vi "AB_1200_1100_Project_Destinations.vi"(6 "ProjectPath":path, 7 "action":T3, 8 "error in (no error)":errorcluster, 9 "index":i32, 10 "data in":T2, 11 "buildObject":T1) -> (0 "error out":errorcluster, 1 "index out":i32, 2 "data out":T2, 3 "buildObject out":T1)   [LabVIEW 2020]
doc: "Reads and writes the data to the object property bag."
uses:
  <resource>/Framework/Providers/API/ItemRef.ctl
  <vilib>/AppBuilder/RW_Project/AB_RW_Project_PropBag_Action.ctl
  <vilib>/AppBuilder/AB_Relative_Path_Type.ctl
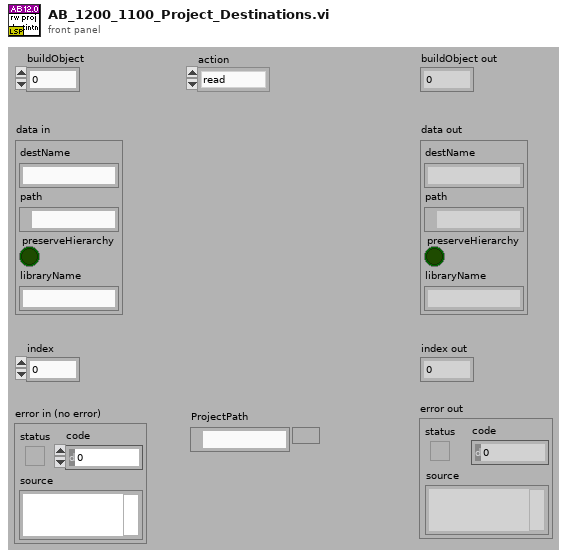
[diagram p1: front panel]
types:
  T1 = typedef "ItemRef.ctl" = u64
  T2 = cluster{"destName":string, "path":path, "preserveHierarchy":bool, "libraryName":string}
  T3 = typedef "AB_RW_Project_PropBag_Action.ctl" = enum16{"read", "write", "clear", "readPrevious", "writePrevious", "clearPrevious"}
  T4 = typedef "AB_Relative_Path_Type.ctl" = enum16{"<none>", "relativeToCommon", "relativeToAppDir", "relativeToProject"}
  T5 = typedef "AB_820_850_Relative_Path_Type.ctl" = enum16{"<none>", "relativeToCommon", "relativeToAppDir"}
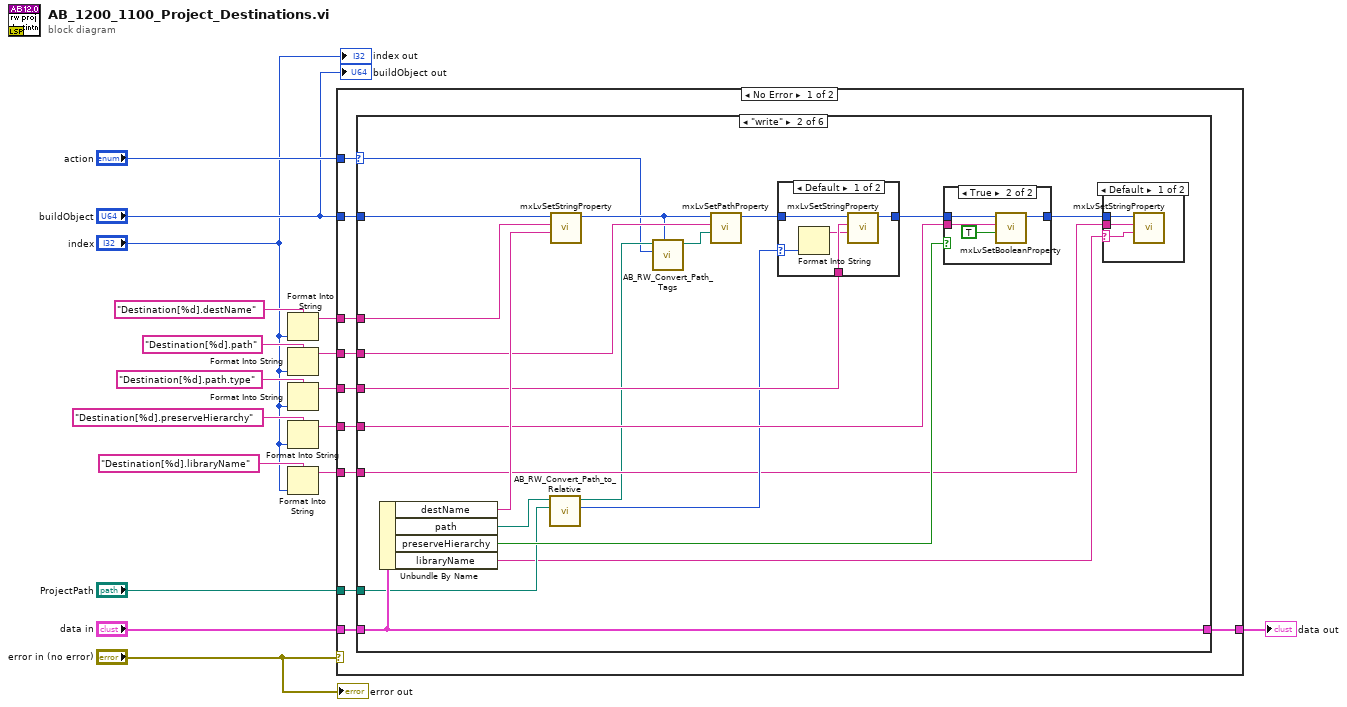
[diagram p0: block diagram]
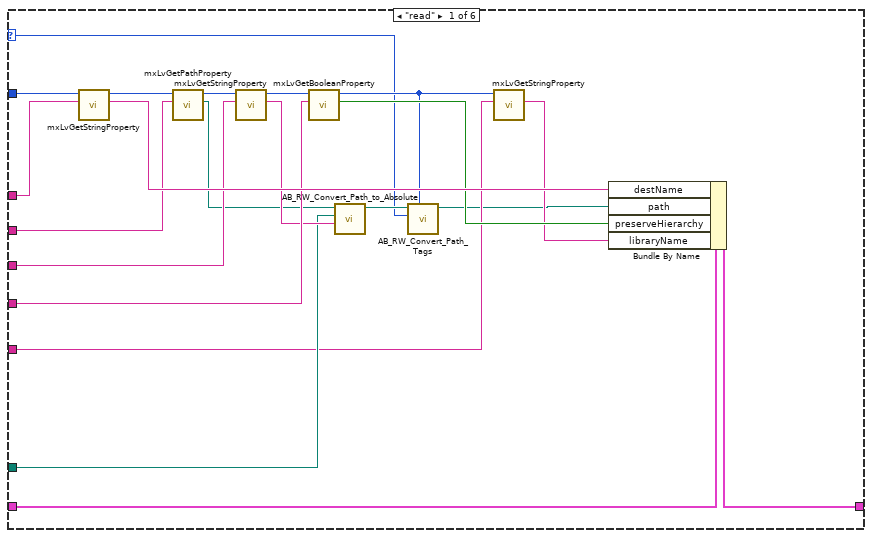
[diagram p2: hidden frame]
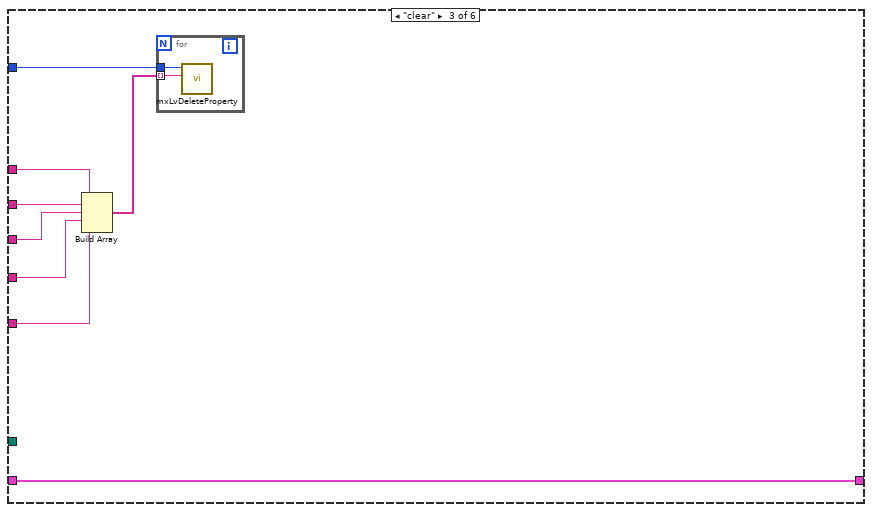
[diagram p6: hidden frame]
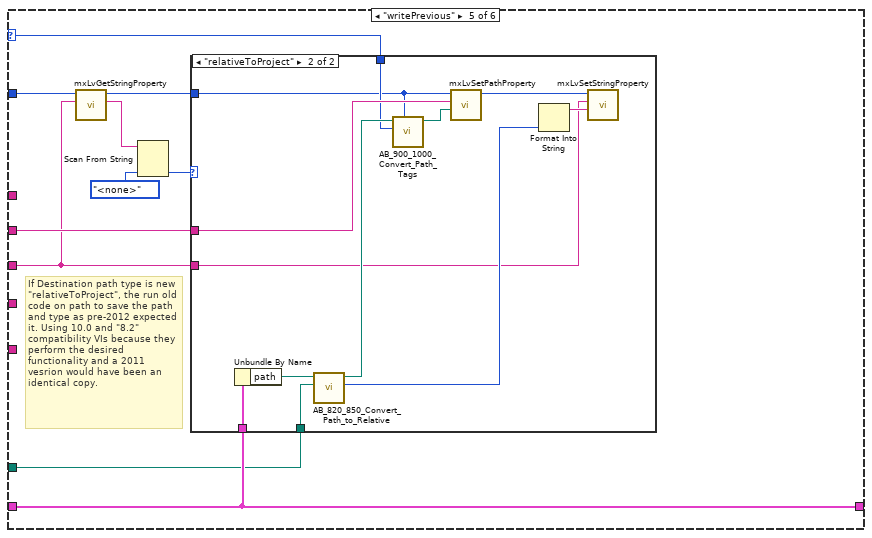
[diagram p8: hidden frame]
diagram:
  n1 = Format Into String(format string="Destination[%d].destName", "index") -> (resulting string=w14:string)  [unwired: 2 in, 1 out]
  n2 = Format Into String(format string="Destination[%d].path", "index") -> (resulting string=w11:string)  [unwired: 2 in, 1 out]
  n3 = Format Into String(format string="Destination[%d].path.type", "index") -> (resulting string=w10:string)  [unwired: 2 in, 1 out]
  n4 = Format Into String(format string="Destination[%d].preserveHierarchy", "index") -> (resulting string=w4:string)  [unwired: 2 in, 1 out]
  n5 = Format Into String(format string="Destination[%d].libraryName", "index") -> (resulting string=w3:string)  [unwired: 2 in, 1 out]
  n6 = case shown="No Error" "error in (no error)" {
    tunnel: "action" -> [w27 _]
    tunnel: "data in" -> [w26 w117]
    tunnel: w14 -> [w25 _]
    tunnel: w11 -> [w24 _]
    tunnel: w10 -> [w23 _]
    tunnel: [w22 w117] -> w9
    tunnel: "buildObject" -> [w21 _]
    tunnel: "ProjectPath" -> [w20 _]
    tunnel: w4 -> [w19 _]
    tunnel: w3 -> [w18 _]
    frame No Error {
      n7 = case shown="\"write\"" w27 {
        selector: w27 -> [w28 w49 _ _ w100 _]
        tunnel: w21 -> [w48 w67 w86 _ w98 _]
        tunnel: w26 -> [w47 w68 w90 w93 w103 w116]
        tunnel: w25 -> [w45 w66 w88 _ _ _]
        tunnel: w24 -> [w41 w64 w89 _ w102 _]
        tunnel: w23 -> [w40 w63 w87 _ w99 _]
        tunnel: [w44 w68 w90 w93 w103 w116] -> w22
        tunnel: w20 -> [w35 w58 _ _ w101 _]
        tunnel: w19 -> [w37 w59 w84 _ _ _]
        tunnel: w18 -> [w32 w55 w83 _ _ _]
        frame "read" {
          n8 = call <resource>:"mxLvGetStringProperty.vi"("Tag"=w45, "Item"=w48) -> ("Value"=w46:string, "Item"=w42:T1)  [unwired: 1 in, 7 out]
          n9 = call <resource>:"mxLvGetPathProperty.vi"("Tag"=w41, "Item"=w42) -> ("Path"=w34:path, "Item"=w43:T1)  [unwired: 2 in, 6 out]
          n10 = call <resource>:"mxLvGetStringProperty.vi"("Tag"=w40, "Item"=w43) -> ("Value"=w36:string, "Item"=w39:T1)  [unwired: 1 in, 7 out]
          n11 = call <resource>:"mxLvGetBooleanProperty.vi"("Tag"=w37, "Item"=w39) -> ("Value"=w38:bool, "Item"=w31:T1)  [unwired: 1 in, 7 out]
          n12 = call <vilib>:"AB_RW_Convert_Path_to_Absolute.vi"("relativeType"=w36, "commonPath"=w35, "relativePath"=w34) -> ("absolute path"=w30:path)  [unwired: 1 in, 7 out]
          n13 = call <vilib>:"AB_RW_Convert_Path_Tags.vi"("buildObject"=w31, "action"=w28, "Path in"=w30) -> ("Path out"=w29:path)  [unwired: 1 in, 7 out]
          n14 = call <resource>:"mxLvGetStringProperty.vi"("Tag"=w32, "Item"=w31) -> ("Value"=w33:string)  [unwired: 1 in, 8 out]
          n15 = Bundle By Name(cluster=w47, "destName"=w46, "path"=w29, "preserveHierarchy"=w38, "libraryName"=w33) -> (w44:T2)
        }
        frame "write" {
          n16 = Unbundle By Name(w68) -> ("destName"=w65:string, "path"=w57:path, "preserveHierarchy"=w60:bool, "libraryName"=w53:string)
          n17 = call <vilib>:"AB_RW_Convert_Path_to_Relative.vi"("commonPath"=w58, "absolutePath"=w57) -> ("relativeType"=w56:T4, "newPath"=w51:path)  [unwired: 1 in, 7 out]
          n18 = call <resource>:"mxLvSetStringProperty.vi"("Value (\"\")"=w65, "Tag"=w66, "Item"=w67) -> ("Item"=w52:T1)  [unwired: 2 in, 6 out]
          n19 = call <vilib>:"AB_RW_Convert_Path_Tags.vi"("buildObject"=w52, "action"=w49, "Path in"=w51) -> ("Path out"=w50:path)  [unwired: 1 in, 7 out]
          n20 = call <resource>:"mxLvSetPathProperty.vi"("Path"=w50, "Tag"=w64, "Item"=w52) -> ("Item"=w62:T1)  [unwired: 2 in, 6 out]
          n21 = case shown="Default" w56 {
            selector: w56 -> [w80 _]
            tunnel: w62 -> [w81 w82]
            tunnel: w63 -> [w79 _]
            tunnel: [w77 w82] -> w61
            frame Default {
              n22 = Format Into String(w80) -> (resulting string=w78:string)  [unwired: 3 in, 1 out]
              n23 = call <resource>:"mxLvSetStringProperty.vi"("Value (\"\")"=w78, "Tag"=w79, "Item"=w81) -> ("Item"=w77:T1)  [unwired: 2 in, 6 out]
            }
            frame "relativeToCommon" {
            }
          }
          n24 = case shown="True" w60 {
            tunnel: w61 -> [w72 w76]
            tunnel: w59 -> [_ w75]
            tunnel: [w72 w73] -> w54
            frame False {
            }
            frame True {
              n25 = call <resource>:"mxLvSetBooleanProperty.vi"("Value (F)"=TRUE, "Tag"=w75, "Item"=w76) -> ("Item"=w73:T1)  [unwired: 2 in, 6 out]
            }
          }
          n26 = case shown="Default" w53 {
            selector: w53 -> [w69 _]
            tunnel: w54 -> [w70 _]
            tunnel: w55 -> [w71 _]
            frame Default {
              n27 = call <resource>:"mxLvSetStringProperty.vi"("Value (\"\")"=w69, "Tag"=w71, "Item"=w70) -> ()  [unwired: 2 in, 7 out]
            }
            frame "" {
            }
          }
        }
        frame "clear" {
          n28 = Build Array(w88, w89, w87, w84, w83) -> (w85:string[])
          n29 = for {
            tunnel: w86 -> [w92]
            tunnel: w85 -> [w91] mode=indexing
            n30 = call <resource>:"mxLvDeleteProperty.vi"("Tag"=w91, "Item"=w92) -> ()  [unwired: 1 in, 9 out]
          }
        }
        frame "readPrevious" {
        }
        frame "writePrevious" {
          # "If Destination path type is new \"relativeToProject\", the run old code on path to save the path and type as pre-2012 expected it. Using 10.0 and \"8.2\" compatibility VIs because they perform the desired functionality and a 2011 vesrion would have been an identical copy."
          n31 = call <resource>:"mxLvGetStringProperty.vi"("Tag"=w99, "Item"=w98) -> ("Value"=w96:string, "Item"=w97:T1)  [unwired: 1 in, 7 out]
          n32 = Scan From String(input string=w96, default 1=AB_Relative_Path_Type."<none>" ("relativeType")) -> (output 1=w95:T4)  [unwired: 3 in, 3 out]
          n33 = case shown="\"relativeToProject\"" w95 {
            tunnel: w103 -> [_ w115]
            tunnel: w102 -> [_ w114]
            tunnel: w101 -> [_ w112]
            tunnel: w100 -> [_ w107]
            tunnel: w99 -> [_ w105]
            tunnel: w97 -> [_ w104]
            frame "<none>", Default {
            }
            frame "relativeToProject" {
              n34 = Unbundle By Name(w115) -> ("path"=w111:path)
              n35 = call <vilib>:"AB_820_850_Convert_Path_to_Relative.vi"("commonPath"=w112, "absolutePath"=w111) -> ("relativeType"=w110:T5, "newPath"=w109:path)  [unwired: 7 in, 1 out]
              n36 = call <vilib>:"AB_900_1000_Convert_Path_Tags.vi"("buildObject"=w104, "action"=w107, "Path in"=w109) -> ("Path out"=w108:path)  [unwired: 7 in, 1 out]
              n37 = call <resource>:"mxLvSetPathProperty.vi"("Path"=w108, "Tag"=w114, "Item"=w104) -> ("Item"=w113:T1)  [unwired: 2 in, 6 out]
              n38 = Format Into String(w110) -> (resulting string=w106:string)  [unwired: 3 in, 1 out]
              n39 = call <resource>:"mxLvSetStringProperty.vi"("Value (\"\")"=w106, "Tag"=w105, "Item"=w113) -> ()  [unwired: 2 in, 7 out]
            }
          }
        }
        frame "clearPrevious" {
        }
      }
    }
    frame Error {
    }
  }
  "data out" <- w9
  "error out" <- "error in (no error)"
  "buildObject out" <- "buildObject"
  "index out" <- "index"
